vi "LWXPS_PositionerPreCorrectorExcitationSignalGet.vi"(0 "XPS Reference IN":refnum<k24>, 7 "Positioner Name":string, 11 "LabVIEW error IN":errorcluster) -> (3 "XPS Reference OUT":refnum<k24>, 4 "Returned error code":i32, 6 "Frequency":dbl, 8 "Amplitude":dbl, 10 "Time":dbl, 14 "LabVIEW error OUT":errorcluster, 15 "XPS Error String":string)   [LabVIEW 2014]
uses:
  D:/XPSQ8_LabView_Library/Development/Source/Dll/Newport.XPS.CommandInterface.dll
  Dll/Newport.XPS.CommandInterface.dll
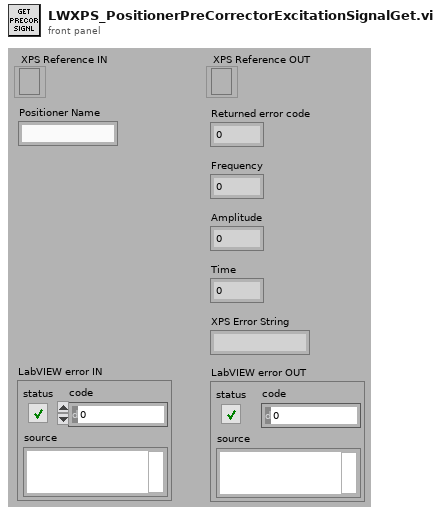
[diagram p1: front panel]
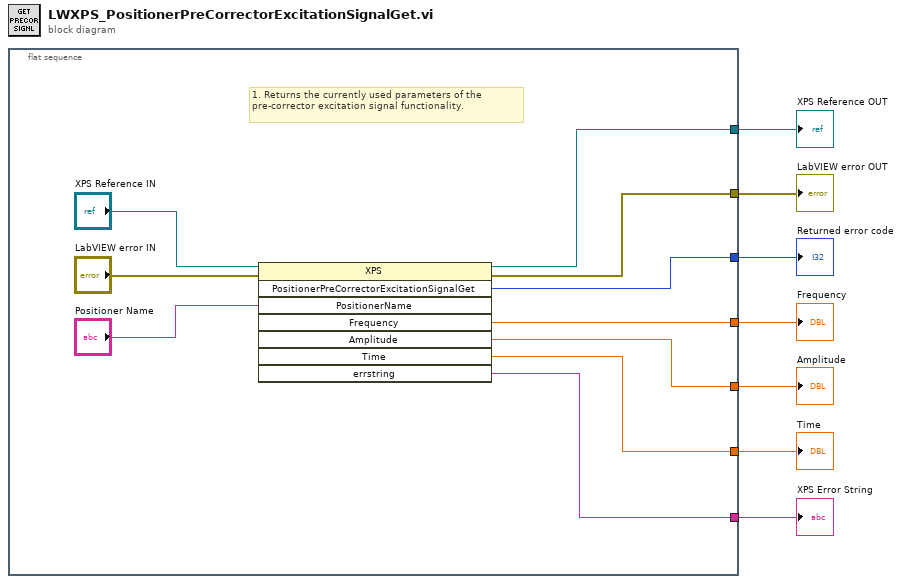
[diagram p0: block diagram]
diagram:
  n1 = flat-sequence {
    tunnel: [w15] -> w7
    tunnel: [w12] -> w6
    tunnel: [w16] -> w5
    tunnel: [w10] -> w2
    tunnel: [w11] -> w4
    tunnel: [w8] -> w3
    tunnel: [w9] -> w1
    frame #0 {
      # "1. Returns the currently used parameters of the pre-corrector excitation signal functionality."
      n2 = invoke class="XPS" method="PositionerPreCorrectorExcitationSignalGet"(reference="XPS Reference IN", error in="LabVIEW error IN", "PositionerName"="Positioner Name") -> (reference out=w15:refnum<k24>, error out=w12:errorcluster, "PositionerPreCorrectorExcitationSignalGet"=w16:i32, "Frequency"=w10:dbl, "Amplitude"=w11:dbl, "Time"=w9:dbl, "errstring"=w8:string)  [unwired: 5 in, 1 out]
    }
  }
  "XPS Error String" <- w3
  "XPS Reference OUT" <- w7
  "LabVIEW error OUT" <- w6
  "Returned error code" <- w5
  "Amplitude" <- w4
  "Frequency" <- w2
  "Time" <- w1
